vi "Scan_Frequency_Range.vi"() -> ()   [LabVIEW 2010]
uses:
  <vilib>/Utility/file.llb/Write To Spreadsheet File (DBL).vi
panel:
  out "Error Phase Shift":cluster{dbl[], dbl[]}(graph)
  out "Error Amplitude":cluster{dbl[], dbl[]}(graph)
  out "Phase Shift":cluster{dbl[], dbl[]}(graph)
  out "Amplitude":cluster{dbl[], dbl[]}(graph)
  in  "Wait [s]":dbl
  in  "Stepsize[Hz]":dbl
  in  "Stop Frequency[Hz]":dbl
  in  "Start Frequency [Hz]":dbl
  out "error out":errorcluster
  in  "error in (no error)":errorcluster
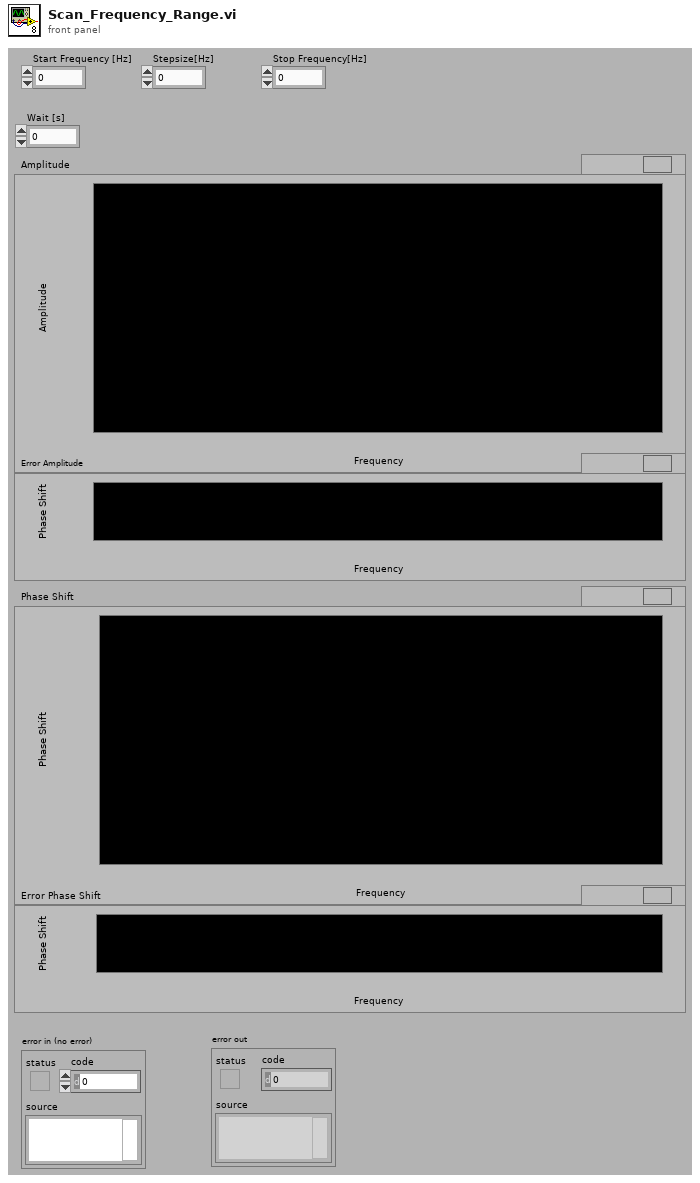
[diagram p1: front panel]
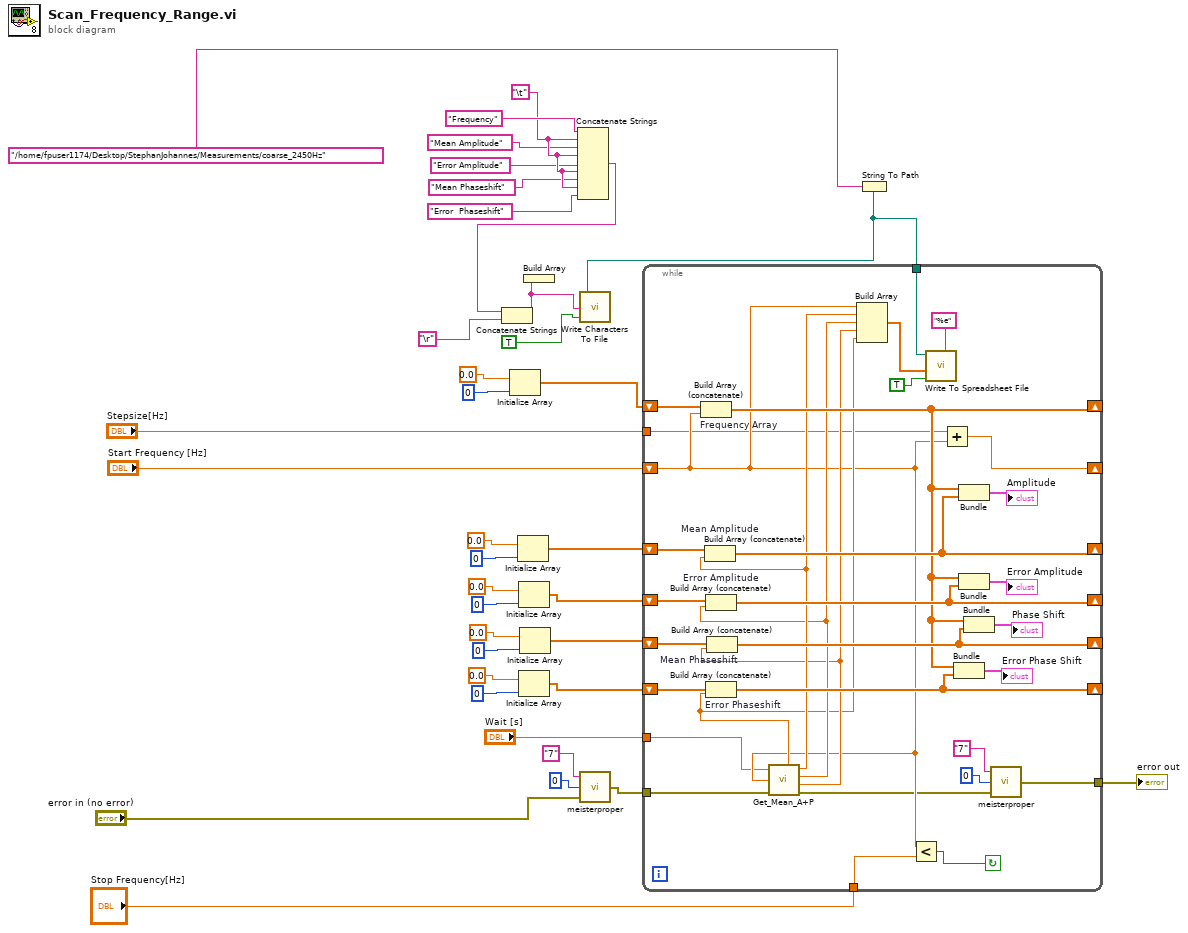
[diagram p0: block diagram]
diagram:
  w27 = "\t"
  n1 = Initialize Array(0.0, 0) -> (w4:dbl[])
  n2 = Initialize Array(0.0, 0) -> (w16:dbl[])
  n3 = Initialize Array(0.0, 0) -> (w9:dbl[])
  n4 = Initialize Array(0.0, 0) -> (w7:dbl[])
  n5 = Initialize Array(0.0, 0) -> (w8:dbl[])
  n6 = Concatenate Strings("Frequency", w27, "Mean Amplitude", w27, "Error Amplitude", w27, "Mean Phaseshift", w27, "Error  Phaseshift") -> (w22:string)
  n7 = Concatenate Strings(w22, "\r") -> (w29:string)
  n8 = Build Array(w29) -> ()  [unwired: 1 out]
  n9 = call "meisterproper.vi"("error in"="error in (no error)", "mode read"=0, "adresse"="7") -> ("error out"=w19:errorcluster)
  n10 = String To Path(string="/home/fpuser1174/Desktop/StephanJohannes/Measurements/coarse_2450Hz") -> (path=w1:path)
  n11 = call <vilib>:"Write Characters To File.vi"("append to file? (new file:F)"=TRUE, "character string"=w29, "file path (dialog if empty)"=w1) -> ()  [unwired: 2 in, 1 out]
  n12 = while {
    tunnel: w19 -> [w43]
    tunnel: [w40] -> w36
    tunnel: "Wait [s]" -> [w38]
    shift-right: [w69] -> _
    shift-left: "Start Frequency [Hz]" -> [w45]
    tunnel: "Stepsize[Hz]" -> [w44]
    tunnel: "Stop Frequency[Hz]" -> [w68]
    shift-right: [w52] -> _
    shift-left: w4 -> [w64]
    shift-right: [w58] -> _
    shift-left: w16 -> [w63]
    shift-right: [w54] -> _
    shift-left: w9 -> [w62]
    shift-right: [w56] -> _
    shift-left: w8 -> [w61]
    shift-right: [w51] -> _
    shift-left: w7 -> [w60]
    tunnel: w1 -> [w37]
    stop <- w67 continue-if-true
    n13 = Build Array (concatenate) "Frequency Array"(w64, w45) -> (w52:dbl[])
    n14 = call "Get_Mean_A+P.vi"("Wait"=w38, "Frequency"=w45, "error in (no error)"=w43) -> ("Mean Amplitude"=w50:dbl, "Error Amplitude"=w49:dbl, "Mean Phase Shift"=w48:dbl, "error out"=w39:errorcluster, "Error Phase Shift"=w47:dbl)
    n15 = Build Array (concatenate) "Mean Amplitude"(w63, w50) -> (w58:dbl[])
    n16 = Build Array (concatenate) "Error Amplitude"(w62, w49) -> (w54:dbl[])
    n17 = Build Array (concatenate) "Error Phaseshift"(w60, w47) -> (w51:dbl[])
    n18 = Build Array (concatenate) "Mean Phaseshift"(w61, w48) -> (w56:dbl[])
    n19 = Build Array(w45, w50, w49, w48, w47) -> (w46:dbl[])
    n20 = Less?(x=w45, y=w68) -> (x < y?=w67:bool)
    n21 = call-poly <vilib>:"Write To Spreadsheet File.vi"("format (%.3f)"="%e", "append to file? (new file:F)"=TRUE, "1D data"=w46, "file path (dialog if empty)"=w37) -> ()  [unwired: 4 in, 1 out]
    n22 = Add(x=w44, y=w45) -> (x+y=w69:dbl)
    n23 = Bundle(w52, w51) -> (→"Error Phase Shift":cluster{dbl[], dbl[]})  [unwired: 1 in]
    n24 = Bundle(w52, w58) -> (→"Amplitude":cluster{dbl[], dbl[]})  [unwired: 1 in]
    n25 = Bundle(w52, w54) -> (→"Error Amplitude":cluster{dbl[], dbl[]})  [unwired: 1 in]
    n26 = Bundle(w52, w56) -> (→"Phase Shift":cluster{dbl[], dbl[]})  [unwired: 1 in]
    n27 = call "meisterproper.vi"("error in"=w39, "mode read"=0, "adresse"="7") -> ("error out"=w40:errorcluster)
  }
  "error out" <- w36
